vi "Open_Create_Replace File.vi"(4 "advisory dialog? (display:T)":bool=TRUE, 5 "pattern":string, 6 "default name":string, 7 "prompt":string, 8 "error in (no error)":errorcluster, 9 "function (open:0)":T2(ring), 10 "start path  (Not A Path)":path=path "", 11 "file path":path) -> (0 "error out":errorcluster, 1 "file size (bytes)":i32, 2 "new file path":path, 3 "refnum":refnum<file>)   [LabVIEW 2013]
doc: "LabVIEW no longer supports this VI. Use the Open/Create/Replace File function instead. Opens an existing file, creates a new file, or replaces an existing file, programmatically or interactively using a file dialog box. You can optionally specify a dialog <B>prompt</B>, default file name, <B>start path</B>, or filter <B>pattern</B>."
panel:
  in  "Messages":T1={"Replace existing \"%s\"?"="Replace existing \"%s\"?", "File \"%s\" exists."="File \"%s\" exists.", "Cancel"="Cancel", "Replace"="Replace", "\"%s\" not found."="\"%s\" not found.", "Open File"="Open File", "New File"="New File", "Create File (file exists)"="Create File (file exists)", "File Dialog"="File Dialog", "Open or Create File %d"="Open or Create File (function=%d)", "EOF"="EOF"}
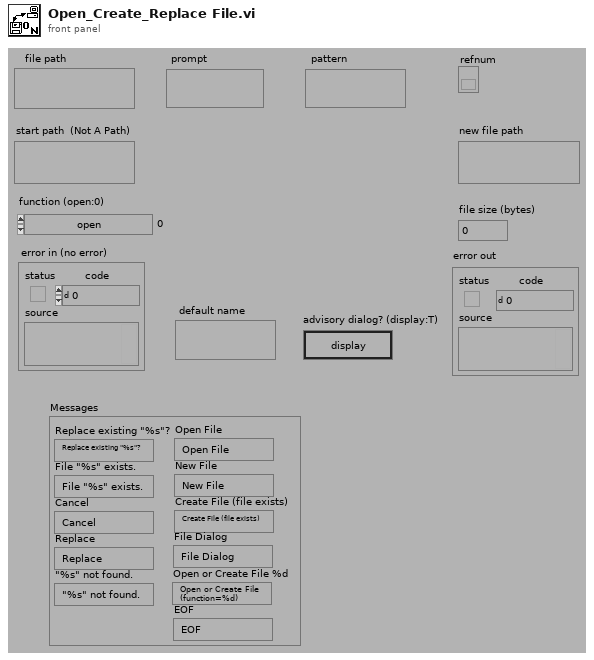
[diagram p1: front panel]
types:
  T1 = cluster{"Replace existing \"%s\"?":string, "File \"%s\" exists.":string, "Cancel":string, "Replace":string, "\"%s\" not found.":string, "Open File":string, "New File":string, "Create File (file exists)":string, "File Dialog":string, "Open or Create File %d":string, "EOF":string}
  T2 = enum16{"open", "open or create", "create or replace", "create", "open (read only)"}
  T3 = enum16{"read/write", "read-only", "write-only", "write-only (truncate)"}
  T4 = enum16{"open", "open or create", "create or replace", "create"}
  T5 = enum16{"existing only", "existing only, truncate", "new only", "new or existing", "new or existing, truncate", "new or existing (confirm dialog)", "new or existing, truncate (confirm dialog)"}
  T6 = enum16{"existing file", "new file", "new or existing file", "existing dir", "new dir", "new or existing dir"}[]
  T7 = enum16{"existing file", "new file", "new or existing file", "existing dir", "new dir", "new or existing dir"}
  T8 = enum16{"open", "replace", "create", "open or create", "replace or create", "replace or create with confirmation"}
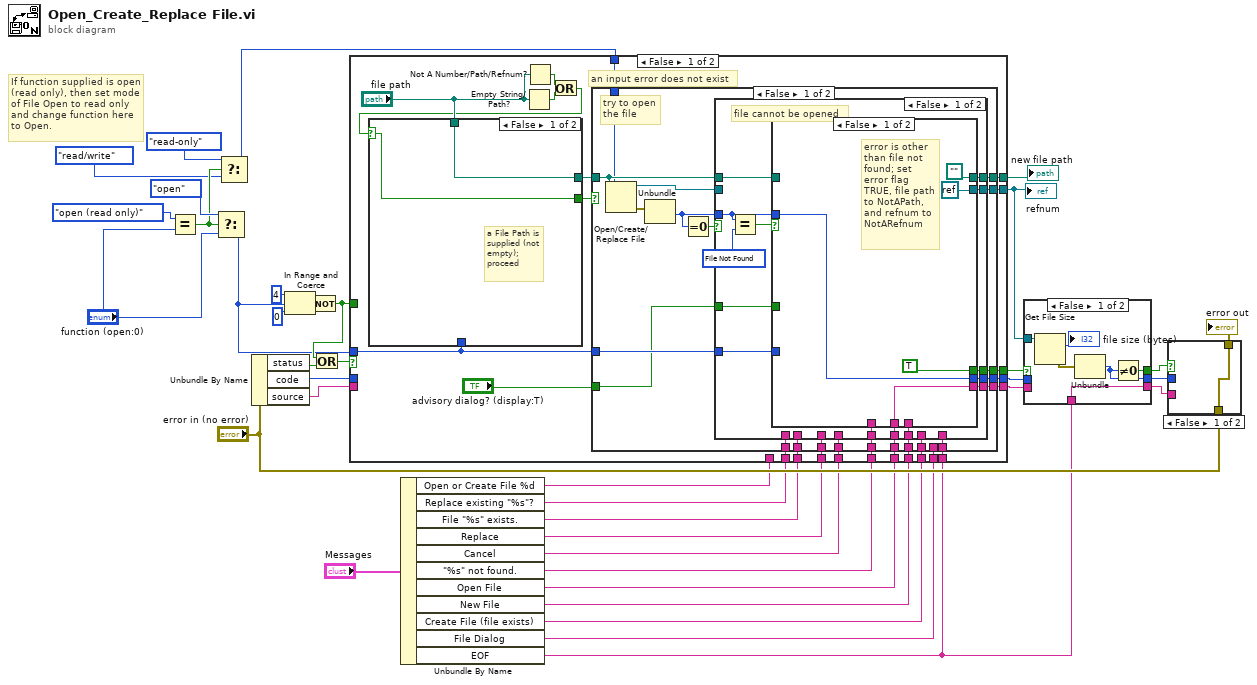
[diagram p0: block diagram]
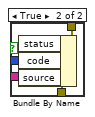
[diagram p2: hidden frame]
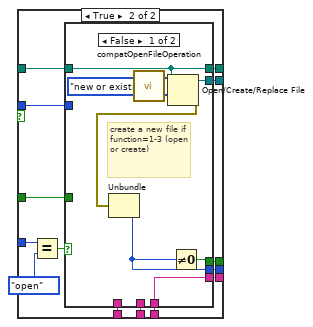
[diagram p4: hidden frame]
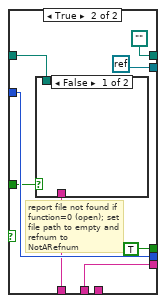
[diagram p5: hidden frame]
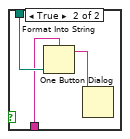
[diagram p6: hidden frame]
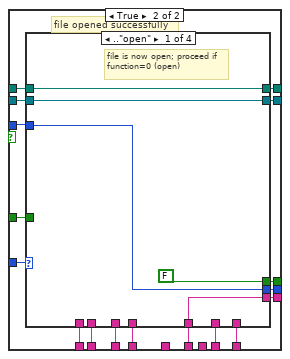
[diagram p7: hidden frame]
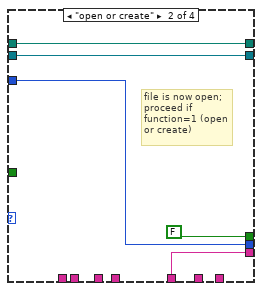
[diagram p8: hidden frame]
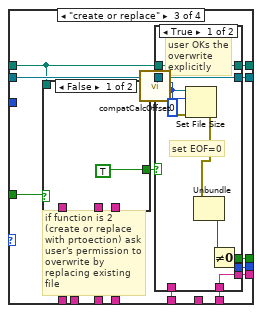
[diagram p9: hidden frame]
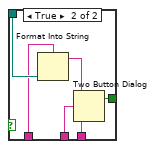
[diagram p10: hidden frame]
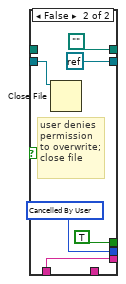
[diagram p11: hidden frame]
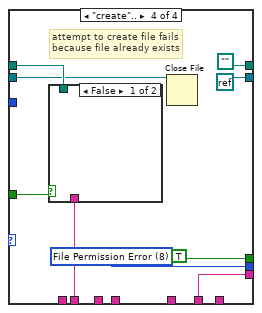
[diagram p12: hidden frame]
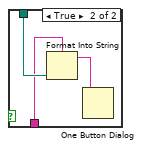
[diagram p13: hidden frame]
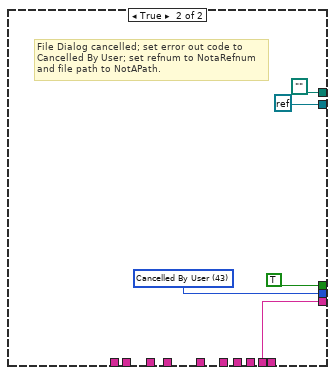
[diagram p14: hidden frame]
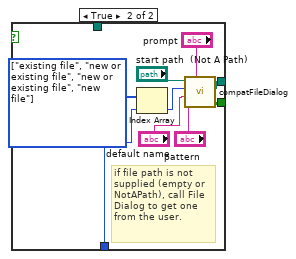
[diagram p15: hidden frame]
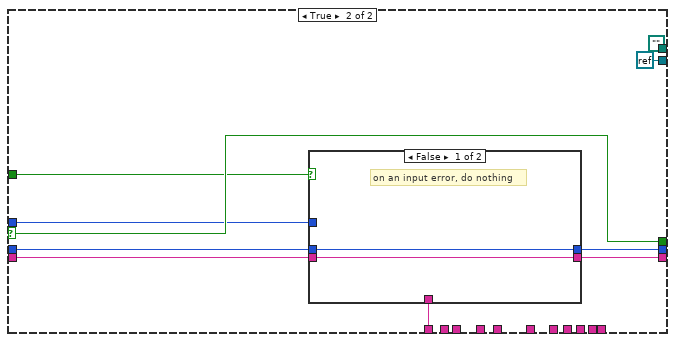
[diagram p16: hidden frame]
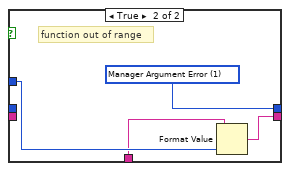
[diagram p17: hidden frame]
diagram:
  # "If function supplied is open (read only), then set mode of File Open to read only and change function here to Open."
  n1 = Equal?(x=T2."open (read only)" ("y"), y="function (open:0)") -> (x = y?=w6:bool)
  n2 = Select(t=T2."open", s=w6, f="function (open:0)") -> (s? t:f=w3:T2)
  n3 = Select(t=T3."read-only" ("open mode (0)"), s=w6, f=T3."read/write" ("open mode (0)")) -> (s? t:f=w1:T3)
  n4 = Unbundle By Name("error in (no error)") -> ("status"=w28:bool, "code"=w27:i32, "source"=w26:string)
  n5 = In Range and Coerce(upper limit=4, x=w3, lower limit=0) -> (In Range?=w33:bool)  [unwired: 1 out]
  n6 = Not(x=w33) -> (.not. x?=w35:bool)
  n7 = Or(x=w35, y=w28) -> (x .or. y?=w34:bool)
  n8 = Unbundle By Name("Messages") -> ("Open or Create File %d"=w10:string, "Replace existing \"%s\"?"=w19:string, "File \"%s\" exists."=w18:string, "Replace"=w17:string, "Cancel"=w16:string, "\"%s\" not found."=w15:string, "Open File"=w14:string, "New File"=w13:string, "Create File (file exists)"=w12:string, "File Dialog"=w11:string, "EOF"=w9:string)
  n9 = case shown="False" w34 {
    selector: w34 -> [_ w236]
    tunnel: [w60 path ""] -> w38
    tunnel: [w59 refnum<k0> refnum] -> w29
    tunnel: [w58 w233] -> w30
    tunnel: [w57 w236] -> w32
    tunnel: [w56 w235] -> w31
    tunnel: w27 -> [_ w234]
    tunnel: w26 -> [_ w232]
    tunnel: w3 -> [w50 w231]
    tunnel: w35 -> [_ w230]
    tunnel: w14 -> [w49 _]
    tunnel: w13 -> [w48 _]
    tunnel: w15 -> [w47 _]
    tunnel: w16 -> [w46 _]
    tunnel: w17 -> [w45 _]
    tunnel: w19 -> [w44 _]
    tunnel: w12 -> [w43 _]
    tunnel: w18 -> [w42 _]
    tunnel: w11 -> [w41 _]
    tunnel: w10 -> [_ w229]
    tunnel: w9 -> [w40 _]
    tunnel: w1 -> [w39 _]
    frame False {
      # "an input error does not exist"
      n10 = Empty String/Path?(string/path="file path") -> (empty?=w53:bool)
      n11 = Not A Number/Path/Refnum?(number/path/refnum="file path") -> (NaN/Path/Refnum?=w54:bool)
      n12 = Or(x=w54, y=w53) -> (x .or. y?=w52:bool)
      n13 = case shown="False" w52 {
        selector: w52 -> [w218 _]
        tunnel: [w218 w226] -> w62
        tunnel: [w219 w225] -> w61
        tunnel: "file path" -> [w219 _]
        tunnel: w50 -> [_ w221]
        frame False {
          # "a File Path is supplied (not empty); proceed"
        }
        frame True {
          w222 = T6 [enum."existing file", enum."new or existing file", enum."new or existing file", enum."new file"] items=["existing file", "new file", "new or existing file", "existing dir", "new dir", "new or existing dir"]
          # "if file path is not supplied (empty or NotAPath), call File Dialog to get one from the user."
          n14 = Index Array(array=w222, index=w221) -> (element=w223:T7)
          n15 = call "compatFileDialog.vi"("prompt"="prompt", "pattern"="pattern", "default name"="default name", "select mode (2)"=w223, "start path"="start path  (Not A Path)") -> ("cancelled"=w226:bool, "path"=w225:path)  [unwired: 4 in, 1 out]
        }
      }
      n16 = case shown="False" w62 {
        tunnel: w61 -> [w83 _]
        tunnel: [w82 path ""] -> w60
        tunnel: w50 -> [w81 _]
        tunnel: [w80 refnum<k0> refnum] -> w59
        tunnel: [w78 w213] -> w58
        tunnel: [w77 TRUE] -> w57
        tunnel: [w76 w216] -> w56
        tunnel: "advisory dialog? (display:T)" -> [w74 _]
        tunnel: w49 -> [w72 _]
        tunnel: w48 -> [w71 _]
        tunnel: w47 -> [w70 _]
        tunnel: w46 -> [w69 _]
        tunnel: w45 -> [w68 _]
        tunnel: w44 -> [w67 _]
        tunnel: w43 -> [w66 _]
        tunnel: w42 -> [w65 _]
        tunnel: w41 -> [_ w213]
        tunnel: w40 -> [w64 _]
        tunnel: w39 -> [w63 _]
        frame False {
          # "try to open the file"
          n17 = Open/Create/Replace File(file path (use dialog)=w83, access (0:read/write)=w63) -> (refnum out=w79:refnum<file>, error out=w84:errorcluster)  [unwired: 4 in, 1 out]
          n18 = Unbundle(w84) -> ("code"=w73:i32)  [unwired: 2 out]
          n19 = Equal To 0?(x=w73) -> (x = 0?=w75:bool)
          n20 = case shown="False" w75 {
            tunnel: w73 -> [w89 w146]
            tunnel: w83 -> [w96 w152]
            tunnel: [w95 w153] -> w82
            tunnel: w81 -> [w94 w145]
            tunnel: [w93 w151] -> w80
            tunnel: w79 -> [_ w150]
            tunnel: [w92 w149] -> w78
            tunnel: [w91 w148] -> w77
            tunnel: [w90 w147] -> w76
            tunnel: w74 -> [w88 w144]
            tunnel: w72 -> [w87 w143]
            tunnel: w71 -> [w86 _]
            tunnel: w70 -> [w85 _]
            tunnel: w69 -> [_ w142]
            tunnel: w68 -> [_ w141]
            tunnel: w67 -> [_ w140]
            tunnel: w66 -> [_ w139]
            tunnel: w65 -> [_ w138]
            tunnel: w64 -> [_ w137]
            frame False {
              w98 = u16 7 items=["No Error", "Manager Argument Error", "Memory Full", "Out of Zone", "End of File", "File Already Open", "Generic File IO Error", "File Not Found", "File Permission Error", "Disk Full", "Duplicate Path", "Too Many Files Open", "Not Enabled", "Resource File Not Found", "Cannot Add Resource", "Resource Not Found", "Image Not Found", "Image Memory Error", "Pen Does Not Exist", "Config Bad Type", "Config Token Not Found", "Config Parse Error", "Config Memory Error", "Bad External Code Format", "Bad External Code Offset", "External Code Not Present", "Null Window", "Destroy Window Mixup", "Null Menu", "Print Aborted", "Bad Print Record", "Print Driver Error", "Windows Error During Print", "Memory Error During Print", "Print Dialog Error", "Generic Print Error", "Invalid Device Refnum", "Device Not Found", "Device Parameter Error", "Device Unit Error", "Can't Open Device", "Device Call Aborted", "Generic Error", "Cancelled By User"]
              # "file cannot be opened"
              n21 = Equal?(x=w89, y=w98) -> (x = y?=w97:bool)
              n22 = case shown="False" w97 {
                tunnel: w96 -> [_ w117]
                tunnel: [path "" w116] -> w95
                tunnel: w94 -> [_ w109]
                tunnel: [refnum<k0> refnum w115] -> w93
                tunnel: [w99 w114] -> w92
                tunnel: [TRUE w113] -> w91
                tunnel: [w100 w112] -> w90
                tunnel: w89 -> [w100 w111]
                tunnel: w88 -> [_ w110]
                tunnel: w87 -> [w99 w105]
                tunnel: w86 -> [_ w106]
                tunnel: w85 -> [_ w104]
                frame False {
                  # "error is other than file not found; set error flag TRUE, file path to NotAPath, and refnum to NotARefnum"
                }
                frame True {
                  n23 = Equal?(x=w109, y=T4."open") -> (x = y?=w108:bool)
                  n24 = case shown="False" w108 {
                    tunnel: w117 -> [w125 w131]
                    tunnel: [w125 path ""] -> w116
                    tunnel: [w124 refnum<k0> refnum] -> w115
                    tunnel: [w120 w127] -> w114
                    tunnel: [w123 TRUE] -> w113
                    tunnel: [w121 w132] -> w112
                    tunnel: w111 -> [_ w132]
                    tunnel: w110 -> [_ w128]
                    tunnel: w106 -> [w120 _]
                    tunnel: w105 -> [_ w127]
                    tunnel: w104 -> [_ w126]
                    frame False {
                      # "create a new file if function=1-3 (open or create)"
                      n25 = call "compatOpenFileOperation.vi"("operation (existing)"=T5."new or existing" ("operation (0:existing only)")) -> ("operation (open)"=w118:T8)
                      n26 = Open/Create/Replace File(file path (use dialog)=w125, operation (0:open)=w118) -> (refnum out=w124:refnum<file>, error out=w122:errorcluster)  [unwired: 4 in, 1 out]
                      n27 = Unbundle(w122) -> ("code"=w121:i32)  [unwired: 2 out]
                      n28 = Not Equal To 0?(x=w121) -> (x != 0?=w123:bool)
                    }
                    frame True {
                      # "report file not found if function=0 (open); set file path to empty and refnum to NotARefnum"
                      n29 = case shown="False" w128 {
                        tunnel: w131 -> [_ w136]
                        tunnel: w126 -> [_ w135]
                        frame False {
                        }
                        frame True {
                          n30 = Format Into String(format string=w135, w136) -> (resulting string=w134:string)  [unwired: 2 in, 1 out]
                          n31 = One Button Dialog(message=w134) -> ()  [unwired: 1 in, 1 out]
                        }
                      }
                    }
                  }
                }
              }
            }
            frame True {
              # "file opened successfully"
              n32 = case shown="..\"open\"" w145 {
                tunnel: [w158 w160 w177 path ""] -> w153
                tunnel: w152 -> [w158 w160 w169 w209]
                tunnel: [w157 w161 w176 refnum<k0> refnum] -> w151
                tunnel: w150 -> [w157 w161 w175 w206]
                tunnel: [w154 w159 w174 w202] -> w149
                tunnel: [FALSE FALSE w173 TRUE] -> w148
                tunnel: [w155 w163 w172 w207] -> w147
                tunnel: w146 -> [w155 w163 _ _]
                tunnel: w144 -> [_ _ w170 w208]
                tunnel: w143 -> [w154 w159 w165 _]
                tunnel: w142 -> [_ _ w168 _]
                tunnel: w141 -> [_ _ w167 _]
                tunnel: w140 -> [_ _ w166 _]
                tunnel: w139 -> [_ _ _ w202]
                tunnel: w138 -> [_ _ _ w201]
                tunnel: w137 -> [_ _ w164 _]
                frame .."open" {
                  # "file is now open; proceed if function=0 (open)"
                }
                frame "open or create" {
                  # "file is now open; proceed if function=1 (open or create)"
                }
                frame "create or replace" {
                  # "if function is 2 (create or replace with prtoection) ask user's permission to overwrite by replacing existing file"
                  n33 = case shown="False" w170 {
                    tunnel: [TRUE w184] -> w171
                    tunnel: w169 -> [_ w181]
                    tunnel: w168 -> [_ w182]
                    tunnel: w167 -> [_ w183]
                    tunnel: w166 -> [_ w179]
                    frame False {
                    }
                    frame True {
                      n34 = Format Into String(format string=w179, w181) -> (resulting string=w180:string)  [unwired: 2 in, 1 out]
                      n35 = Two Button Dialog(message=w180, 1:w182, 2:w183) -> (T button?=w184:bool)
                    }
                  }
                  n36 = case shown="True" w171 {
                    tunnel: [w190 path ""] -> w177
                    tunnel: [w194 refnum<k0> refnum] -> w176
                    tunnel: w175 -> [w194 w198]
                    tunnel: [w188 w195] -> w174
                    tunnel: [w192 TRUE] -> w173
                    tunnel: [w189 w196] -> w172
                    tunnel: w169 -> [w190 _]
                    tunnel: w165 -> [_ w195]
                    tunnel: w164 -> [w188 _]
                    frame True {
                      w193 = 0
                      # "set EOF=0"
                      # "user OKs the overwrite explicitly"
                      n37 = call "compatCalcOffset.vi"("pos offset (0)"=w193, "pos mode (0:1)"=w193, "refnum"=w194) -> ("error out"=w187:errorcluster, "offset"=w186:i32, "dup refnum"=w185:refnum<file>)  [unwired: 6 in]
                      n38 = Set File Size(4:w187, 6:w186, 7:w185) -> (0:w191:errorcluster)  [unwired: 1 out]
                      n39 = Unbundle(w191) -> ("code"=w189:i32)  [unwired: 2 out]
                      n40 = Not Equal To 0?(x=w189) -> (x != 0?=w192:bool)
                    }
                    frame False {
                      w196 = u16 43 items=["No Error", "Manager Argument Error", "Memory Full", "Out of Zone", "End of File", "File Already Open", "Generic File IO Error", "File Not Found", "File Permission Error", "Disk Full", "Duplicate Path", "Too Many Files Open", "Not Enabled", "Resource File Not Found", "Cannot Add Resource", "Resource Not Found", "Image Not Found", "Image Memory Error", "Pen Does Not Exist", "Config Bad Type", "Config Token Not Found", "Config Parse Error", "Config Memory Error", "Bad External Code Format", "Bad External Code Offset", "External Code Not Present", "Null Window", "Destroy Window Mixup", "Null Menu", "Print Aborted", "Bad Print Record", "Print Driver Error", "Windows Error During Print", "Memory Error During Print", "Print Dialog Error", "Generic Print Error", "Invalid Device Refnum", "Device Not Found", "Device Parameter Error", "Device Unit Error", "Can't Open Device", "Device Call Aborted", "Generic Error", "Cancelled By User"]
                      # "user denies permission to overwrite; close file"
                      n41 = Close File(refnum=w198) -> ()  [unwired: 1 in, 2 out]
                    }
                  }
                }
                frame "create".. {
                  w207 = u16 8 items=["No Error", "Argument Error", "Memory Full", "Out of Zone", "End of File", "File Already Open", "Generic File IO Error", "File Not Found", "File Permission Error", "Disk Full", "Duplicate Path", "Too Many Files Open", "Not Enabled", "Resource File Not Found", "Cannot Add Resource", "Resource Not Found", "Image Not Found", "Image Memory Error", "Pen Does Not Exist", "Config Bad Type", "Config Token Not Found", "Config Parse Error", "Config Memory Error", "Bad External Code Format", "Bad External Code Offset", "External Code Not Present", "Null Window", "Destroy Window Mixup", "Null Menu", "Print Aborted", "Bad Print Record", "Print Driver Error", "Windows Error During Print", "Memory Error During Print", "Print Dialog Error", "Generic Print Error", "Invalid Device Refnum", "Device Not Found", "Device Parameter Error", "Device Unit Error", "Can't Open Device", "Device Call Aborted", "Generic Error", "Cancelled By User", "Object ID Too Low", "Object ID Too High", "Object Not In Heap", "Unknown Heap", "Bad DefProc ID", "DefProc Not In Table", "Message Out Of Range", "Null Method", "Unknown Message", "Manager Call Not Supported", "Bad address", "Connection In progress", "Connection timed out", "Connection is already in progress", "Network attribute not supported", "Network error", "Address in use", "System out of memory", "Connection aborted", "Connection refused", "Connection is not connected", "Connection is already connected", "Connection closed", "Initialize error (interapplication manager)", "Bad occurrence", "Wait on unbound occurrence handler", "Occurrence queue overflow", "Bad path", "Semaphore not signaled", "Unrecognized type (interapplication manager)"]
                  # "attempt to create file fails because file already exists"
                  n42 = case shown="False" w208 {
                    tunnel: w209 -> [_ w212]
                    tunnel: w201 -> [_ w210]
                    frame False {
                    }
                    frame True {
                      n43 = Format Into String(format string=w210, w212) -> (resulting string=w211:string)  [unwired: 2 in, 1 out]
                      n44 = One Button Dialog(message=w211) -> ()  [unwired: 1 in, 1 out]
                    }
                  }
                  n45 = Close File(refnum=w206) -> ()  [unwired: 1 in, 2 out]
                }
              }
            }
          }
        }
        frame True {
          w216 = u16 43 items=["No Error", "Manager Argument Error", "Memory Full", "Out of Zone", "End of File", "File Already Open", "Generic File IO Error", "File Not Found", "File Permission Error", "Disk Full", "Duplicate Path", "Too Many Files Open", "Not Enabled", "Resource File Not Found", "Cannot Add Resource", "Resource Not Found", "Image Not Found", "Image Memory Error", "Pen Does Not Exist", "Config Bad Type", "Config Token Not Found", "Config Parse Error", "Config Memory Error", "Bad External Code Format", "Bad External Code Offset", "External Code Not Present", "Null Window", "Destroy Window Mixup", "Null Menu", "Print Aborted", "Bad Print Record", "Print Driver Error", "Windows Error During Print", "Memory Error During Print", "Print Dialog Error", "Generic Print Error", "Invalid Device Refnum", "Device Not Found", "Device Parameter Error", "Device Unit Error", "Can't Open Device", "Device Call Aborted", "Generic Error", "Cancelled By User"]
          # "File Dialog cancelled; set error out code to Cancelled By User; set refnum to NotaRefnum and file path to NotAPath."
        }
      }
    }
    frame True {
      n46 = case shown="False" w230 {
        tunnel: [w240 w244] -> w235
        tunnel: w234 -> [w240 _]
        tunnel: [w239 w243] -> w233
        tunnel: w232 -> [w239 _]
        tunnel: w231 -> [_ w242]
        tunnel: w229 -> [_ w241]
        frame False {
          # "on an input error, do nothing"
        }
        frame True {
          w244 = u16 1 items=["No Error", "Manager Argument Error", "Memory Full", "Out of Zone", "End of File", "File Already Open", "Generic File IO Error", "File Not Found", "File Permission Error", "Disk Full", "Duplicate Path", "Too Many Files Open", "Not Enabled", "Resource File Not Found", "Cannot Add Resource", "Resource Not Found", "Image Not Found", "Image Memory Error", "Pen Does Not Exist", "Config Bad Type", "Config Token Not Found", "Config Parse Error", "Config Memory Error", "Bad External Code Format", "Bad External Code Offset", "External Code Not Present", "Null Window", "Destroy Window Mixup", "Null Menu", "Print Aborted", "Bad Print Record", "Print Driver Error", "Windows Error During Print", "Memory Error During Print", "Print Dialog Error", "Generic Print Error", "Invalid Device Refnum", "Device Not Found", "Device Parameter Error", "Device Unit Error", "Can't Open Device", "Device Call Aborted", "Generic Error", "Cancelled By User"]
          # "function out of range"
          n47 = Format Value(format string=w241, value (0)=w242) -> (output string=w243:string)  [unwired: 1 in]
        }
      }
    }
  }
  "new file path" <- w38
  "refnum" <- w29
  n48 = case shown="False" w32 {
    selector: w32 -> [_ w253]
    tunnel: w31 -> [_ w252]
    tunnel: w30 -> [_ w251]
    tunnel: [w250 w253] -> w25
    tunnel: [w247 w252] -> w24
    tunnel: [w245 w251] -> w23
    tunnel: w29 -> [w249 _]
    tunnel: w9 -> [w245 _]
    frame False {
      n49 = Get File Size(file=w249) -> (size (in bytes)=→"file size (bytes)":i64, 0:w246:errorcluster)  [unwired: 1 in, 1 out]
      n50 = Unbundle(w246) -> ("code"=w247:i32)  [unwired: 2 out]
      n51 = Not Equal To 0?(x=w247) -> (x != 0?=w250:bool)
    }
    frame True {
    }
  }
  n52 = case shown="False" w25 {
    selector: w25 -> [_ w258]
    tunnel: w24 -> [_ w259]
    tunnel: w23 -> [_ w257]
    tunnel: "error in (no error)" -> [w254 w256]
    tunnel: [w254 w255] -> w21
    frame False {
    }
    frame True {
      n53 = Bundle By Name(cluster=w256, "status"=w258, "code"=w259, "source"=w257) -> (w255:errorcluster)
    }
  }
  "error out" <- w21
